vi "Configure Output Parameters 1.vi"(0 "VISA resource name":refnum<visa-resource-name>, 1 "Unit Address (1)":u8=1, 5 "Channel 2 Deadband (0)":sgl min=0 max=100 format="%.1g", 7 "Output Rate Limit (0)":u16, 9 "Channel 1 Travel Time (0)":sgl min=0 max=1000 format="%.1g", 11 "error in (no error)":errorcluster, 12 "Channel 1 Valve Position (0)":i32, 13 "Channel 1 Potentiometer Break (False)":bool) -> (4 "VISA resource name out":refnum<visa-resource-name>, 15 "error out":errorcluster)   [LabVIEW 2014, in "Eurotherm 35xx Series.lvlib"]
doc: "This VI sets Output Parameters."
uses:
  <instrlib>/Eurotherm 35xx Series/Eurotherm 35xx Series.lvlib
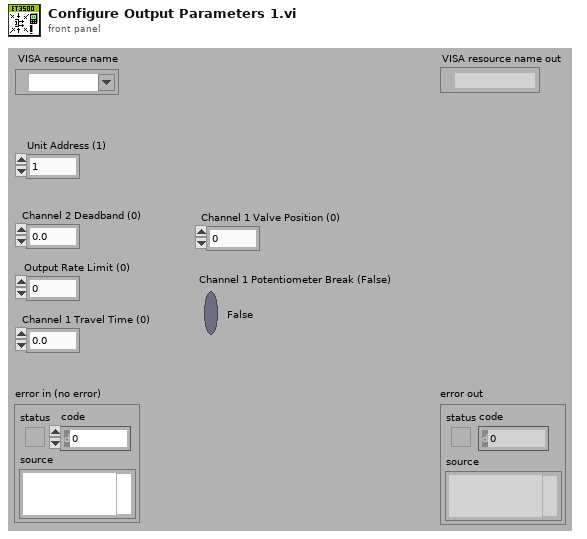
[diagram p1: front panel]
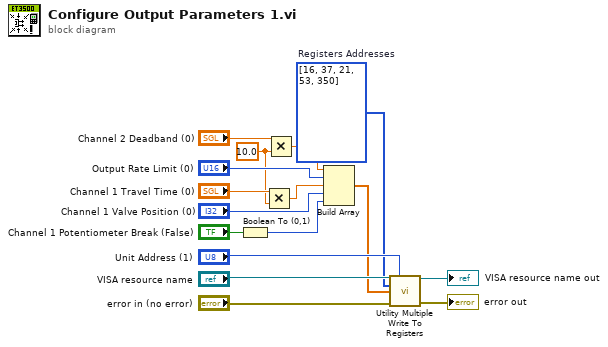
[diagram p0: block diagram]
diagram:
  w3 = sgl 10.0 ("y")
  w8 = u16[] [16, 37, 21, 53, 350]  # Registers Addresses
  n1 = Boolean To (0,1)(Boolean="Channel 1 Potentiometer Break (False)") -> (0, 1=w1:i16)
  n2 = Multiply(x="Channel 1 Travel Time (0)", y=w3) -> (x*y=w4:sgl)
  n3 = Multiply(x="Channel 2 Deadband (0)", y=w3) -> (x*y=w6:sgl)
  n4 = Build Array(w6, "Output Rate Limit (0)", w4, "Channel 1 Valve Position (0)", w1) -> (w9:sgl[])
  n5 = call <instrlib>:"Utility Multiple Write To Registers.vi"("VISA resource name"="VISA resource name", "Unit Address (1)"="Unit Address (1)", "Registers Addresses (0)"=w8, "Data (0)"=w9, "error in (no error)"="error in (no error)") -> ("VISA resource name out"=→"VISA resource name out":refnum<visa-resource-name>, "error out"=→"error out":errorcluster)  [unwired: 9 in]
